vi "在表格前面插入列.vi"(8 "错误输入（无错误）":errorcluster, 10 "内容":string[](array[string]), 11 "引用输入":refnum<vi>) -> (0 "错误输出":errorcluster, 3 "引用输出":refnum<vi>)   [LabVIEW 2014, in "表格.lvlib"]
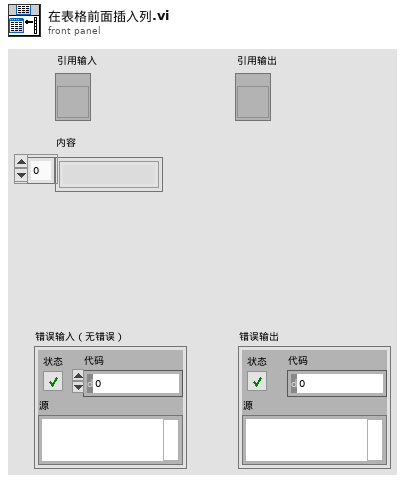
[diagram p1: front panel]
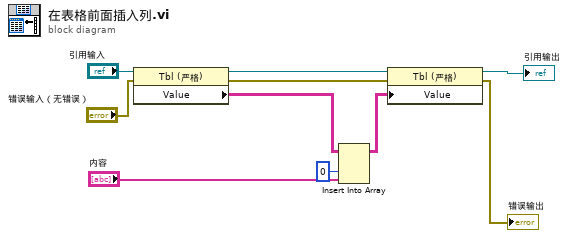
[diagram p0: block diagram]
diagram:
  n1 = property class="Tbl (严格)"(reference="引用输入", error in="错误输入（无错误）") -> (reference out=w10:refnum<vi>, error out=w9:errorcluster, "Value"=w4:string[][])
  n2 = Insert Into Array(array=w4, index (col)=0 ("禁用的索引 (列)"), new element="内容") -> (w2:string[][])  [unwired: 1 in]
  n3 = property class="Tbl (严格)"(reference=w10, error in=w9, "Value"=w2) -> (reference out=→"引用输出":refnum<vi>, error out=→"错误输出":errorcluster)
